vi "Valid.vi"(8 "error in (no error)":errorcluster, 11 "BluePlotHandle in":refnum<class "RocketPlotHandle.lvclass">) -> (0 "error out":errorcluster, 2 "Valid?":bool, 3 "BluePlotHandle out":refnum<class "RocketPlotHandle.lvclass">)   [LabVIEW 2021, in "RocketPlotHandle.lvclass"]
doc: "This returns TRUE if the handle is still valid.\n\nA handle is valid if the plot instance queue reference is still valid.\nA plot instance will destroy the queue instance when it is shutdown."
uses:
  RocketPlotHandle.lvclass
  RocketPlotHandle.lvclass/RocketPlotHandle.ctl
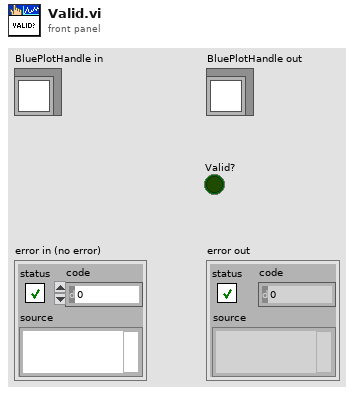
[diagram p1: front panel]
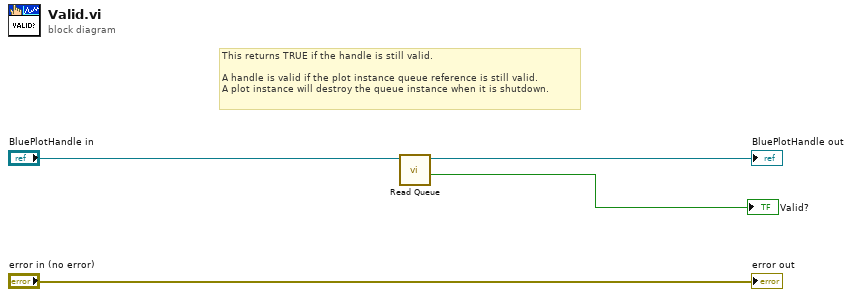
[diagram p0: block diagram]
diagram:
  # "This returns TRUE if the handle is still valid.\n\nA handle is valid if the plot instance queue reference is still valid.\nA plot instance will destroy the queue instance when it is shutdown."
  n1 = call "Read Queue.vi"("BluePlotHandle in"="BluePlotHandle in") -> ("Valid?"=→"Valid?":bool, "BluePlotHandle out"=→"BluePlotHandle out":refnum<class "RocketPlotHandle.lvclass">)  [unwired: 8 in, 1 out]
  "error out" <- "error in (no error)"
